vi "Win Host - Find Short-Cut.vi"(11 "Language in":string) -> (1 "Short-Cut?":bool, 2 "S/CUT Index":i32, 3 "Language out":string)   [LabVIEW 2024]
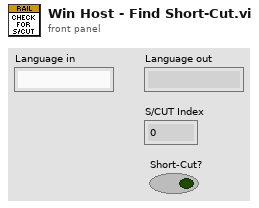
[diagram p1: front panel]
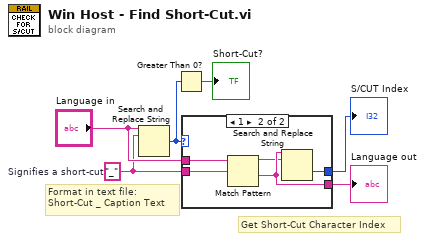
[diagram p0: block diagram]
diagram:
  w1 = "_"  # Signifies a short-cut
  # "Get Short-Cut Character Index"
  # "Format in text file:\nShort-Cut _ Caption Text"
  n1 = Search and Replace String(input string="Language in", search string=w1) -> (number of replacements=w4:i32)  [unwired: 6 in, 3 out]
  n2 = Greater Than 0?(x=w4) -> (x > 0?=→"Short-Cut?":bool)
  n3 = case shown="1" w4 {
    tunnel: w1 -> [_ w12]
    tunnel: "Language in" -> [w7 w11]
    tunnel: [w7 w10] -> w3
    tunnel: [_ w8] -> w5
    frame 0, Default {
      # "No Short-Cut"
    }
    frame 1 {
      n4 = Match Pattern(string=w11, regular expression=w12) -> (before substring=w9:string, after substring=w10:string)  [unwired: 1 in, 2 out]
      n5 = Search and Replace String(input string=w10, search string=w9) -> (offset past replacement=w8:i32)  [unwired: 6 in, 3 out]
    }
  }
  "S/CUT Index" <- w5
  "Language out" <- w3
